vi "Process Telemetry Folder.vi"() -> ()   [LabVIEW 2014]
panel:
  in  "Output Folder":path=path "Y:/Dropbox/Formula Electric 2014-2015/Testing/6-17-15/Intermediate"
  in  "Input Folder":path=path "Y:/Dropbox/Formula Electric 2014-2015/Testing/6-17-15/Unprocessed"
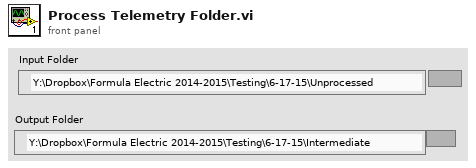
[diagram p1: front panel]
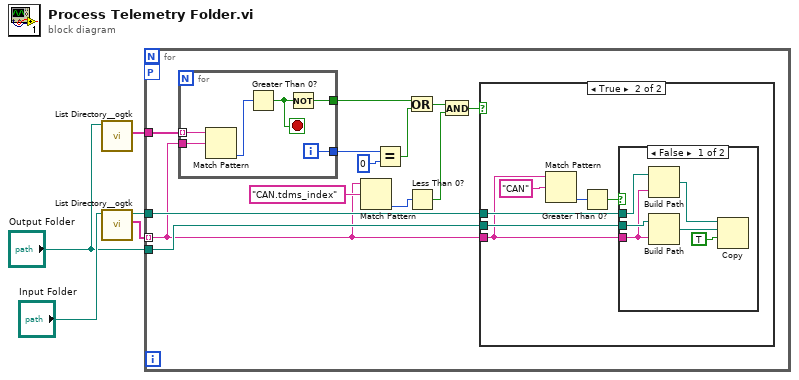
[diagram p0: block diagram]
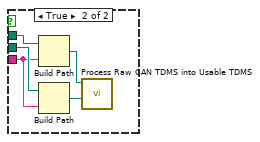
[diagram p3: hidden frame]
diagram:
  n1 = call <userlib>:"List Directory__ogtk.vi"("directory path"="Output Folder") -> ("file names"=w1:string[])  [unwired: 3 in, 3 out]
  n2 = call <userlib>:"List Directory__ogtk.vi"("directory path"="Input Folder") -> ("file names"=w4:string[], "dup directory path"=w3:path)  [unwired: 3 in, 2 out]
  n3 = for {
    tunnel: w4 -> [w11] mode=indexing
    tunnel: w3 -> [w18]
    tunnel: "Output Folder" -> [w17]
    tunnel: w1 -> [w12]
    workers-P: _ -> [_]
    n4 = for {
      tunnel: w12 -> [w24] mode=indexing
      tunnel: [w20] -> w7
      tunnel: w11 -> [w22]
      tunnel: [w19] -> w10
      i -> [w19]
      stop <- w21 stop-if-true
      n5 = Match Pattern(string=w24, regular expression=w22) -> (offset past match=w23:i32)  [unwired: 1 in, 3 out]
      n6 = Greater Than 0?(x=w23) -> (x > 0?=w21:bool)
      n7 = Not(x=w21) -> (.not. x?=w20:bool)
    }
    n8 = Match Pattern(string=w11, regular expression="CAN.tdms_index") -> (offset past match=w15:i32)  [unwired: 1 in, 3 out]
    n9 = Equal?(x=w10, y=0) -> (x = y?=w6:bool)
    n10 = Or(x=w7, y=w6) -> (x .or. y?=w8:bool)
    n11 = Less Than 0?(x=w15) -> (x < 0?=w14:bool)
    n12 = And(x=w8, y=w14) -> (x .and. y?=w13:bool)
    n13 = case shown="True" w13 {
      tunnel: w18 -> [_ w30]
      tunnel: w17 -> [_ w29]
      tunnel: w11 -> [_ w28]
      frame False {
      }
      frame True {
        n14 = Match Pattern(string=w28, regular expression="CAN") -> (offset past match=w26:i32)  [unwired: 1 in, 3 out]
        n15 = Greater Than 0?(x=w26) -> (x > 0?=w25:bool)
        n16 = case shown="False" w25 {
          tunnel: w30 -> [w36 w41]
          tunnel: w29 -> [w35 w39]
          tunnel: w28 -> [w34 w38]
          frame False {
            n17 = Build Path(base path=w36, name or relative path=w34) -> (appended path=w33:path)
            n18 = Build Path(base path=w35, name or relative path=w34) -> (appended path=w32:path)
            n19 = Copy(9:TRUE ("overwrite (F)"), 10:w32, 11:w33) -> ()  [unwired: 2 in, 3 out]
          }
          frame True {
            n20 = Build Path(base path=w41, name or relative path=w38) -> (appended path=w40:path)
            n21 = Build Path(base path=w39, name or relative path=w38) -> (appended path=w37:path)
            n22 = call "Process Raw CAN TDMS into Usable TDMS.vi"("Destination"=w37, "Source"=w40) -> ()  [unwired: 10 in]
          }
        }
      }
    }
  }
